vi "FileIO - Create ALL Directories and Init Reads.vi"(7 "error in":errorcluster) -> (0 "error out":errorcluster)   [LabVIEW 2014]
doc: "Queue Reference:\n\nDefines name queue references for each of the queued state machines. This includes a custom control for both the queue data type (cluster) and a custer of all the queue refnums."
uses:
  TypeDef - Directory Structures.ctl
  TypeDef - File Actions.ctl
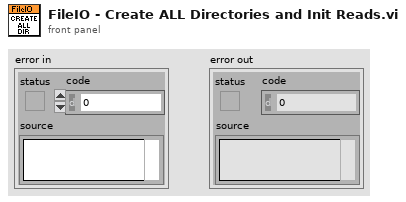
[diagram p1: front panel]
types:
  T1 = typedef "TypeDef - Directory Structures.ctl" = enum16{"Project", "config", "testconfig", "raw data"}
  T2 = typedef "TypeDef - File Actions.ctl" = enum16{"Read", "Write", "Get Current"}
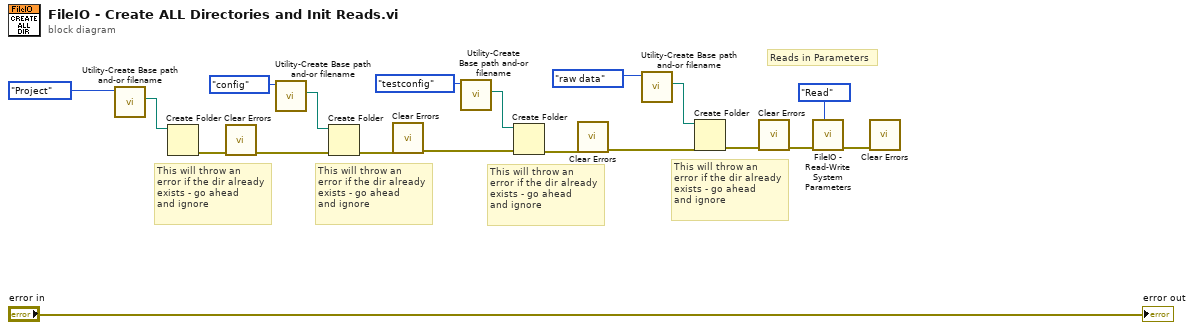
[diagram p0: block diagram]
diagram:
  # "This will throw an\nerror if the dir already\nexists - go ahead\nand ignore"
  # "Reads in Parameters"
  # "This will throw an\nerror if the dir already\nexists - go ahead\nand ignore"
  # "This will throw an\nerror if the dir already\nexists - go ahead\nand ignore"
  # "This will throw an\nerror if the dir already\nexists - go ahead\nand ignore"
  n1 = call "Utility-Create Base path and-or filename.vi"("Directory Name"=TypeDef_-_Directory_Structures."Project") -> ("File name and path"=w17:path)  [unwired: 10 in]
  n2 = Create Folder(path (use dialog)=w17) -> (error out=w16:errorcluster)  [unwired: 2 in, 2 out]
  n3 = call <vilib>:"Clear Errors.vi"("error in (no error)"=w16) -> ("error out"=w13:errorcluster)  [unwired: 5 in, 1 out]
  n4 = call "Utility-Create Base path and-or filename.vi"("Directory Name"=TypeDef_-_Directory_Structures."config") -> ("File name and path"=w15:path)  [unwired: 10 in]
  n5 = Create Folder(path (use dialog)=w15, error in=w13) -> (error out=w12:errorcluster)  [unwired: 1 in, 2 out]
  n6 = call <vilib>:"Clear Errors.vi"("error in (no error)"=w12) -> ("error out"=w4:errorcluster)  [unwired: 5 in, 1 out]
  n7 = call "Utility-Create Base path and-or filename.vi"("Directory Name"=TypeDef_-_Directory_Structures."testconfig") -> ("File name and path"=w5:path)  [unwired: 10 in]
  n8 = Create Folder(path (use dialog)=w5, error in=w4) -> (error out=w3:errorcluster)  [unwired: 1 in, 2 out]
  n9 = call <vilib>:"Clear Errors.vi"("error in (no error)"=w3) -> ("error out"=w2:errorcluster)  [unwired: 5 in, 1 out]
  n10 = call "Utility-Create Base path and-or filename.vi"("Directory Name"=TypeDef_-_Directory_Structures."raw data") -> ("File name and path"=w9:path)  [unwired: 10 in]
  n11 = Create Folder(path (use dialog)=w9, error in=w2) -> (error out=w10:errorcluster)  [unwired: 1 in, 2 out]
  n12 = call <vilib>:"Clear Errors.vi"("error in (no error)"=w10) -> ("error out"=w7:errorcluster)  [unwired: 5 in, 1 out]
  n13 = call "FileIO - Read-Write System Parameters.vi"("Action"=TypeDef_-_File_Actions."Read", "error in (no error)"=w7) -> ("error out"=w1:errorcluster)  [unwired: 8 in, 1 out]
  n14 = call <vilib>:"Clear Errors.vi"("error in (no error)"=w1) -> ()  [unwired: 5 in, 2 out]
  "error out" <- "error in"
